vi "Generation Stream Control (Real 16 SPC).vi"(0 "data in":fxp<+/-,18,1>[](array[numeric])=[0.0, 0.0, 0.0, 0.0, 0.0, 0.0, 0.0, 0.0, 0.0, 0.0, 0.0, 0.0, 0.0, 0.0, 0.0, 0.0], 1 "input valid":bool, 2 "request state":T1, 3 "num samples":u64, 4 "initial padding":u64, 5 "final padding":u64, 7 "ready for output (T)":bool=TRUE, 8 "reset":bool, 9 "start trigger":bool) -> (11 "ready for start":bool, 12 "metadata":u64, 13 "ready for input":bool, 14 "data out":fxp<+/-,18,1>[](array[numeric]), 15 "output valid":bool, 16 "actual state":T1, 17 "samples transferred":u64)   [LabVIEW 2018, in "Streaming FPGA.lvlib"]
doc: "<B>General</B>\n\nThis VI controls the signal generation data flow with a state machine controller. This enables the control and monitoring of finite and continuous streams of data between nodes using 4-wire handshaking.\n\n<B>Signals</B>\n\nThe stream is controlled by the <B>request state</B>, <B>num samples</B>, <B>initial padding</B>, <B>final padding</B> and <B>start trigger</B> inputs. The stream is monitored by the <B>actual state</B>, <B>ready for start</B> and <B>samples transferred</B> outputs. In addition, <b>metadata</b> is available for publishing details about the form/function of the stream.\n\nThe upstream node can provide data on the <B>data in</B> input by setting the <B>input valid</B> input to true. The data provided on the <B>data in</B> input is accepted if the <B>input valid</B> input is true and the <B>ready for input</B> output was true in the previous cycle. If the <B>ready for input</B> output was false in the previous cycle, then the <B>data in</B> and <B>input valid</B> inputs are ignored in the current cycle.\n\nThe <B>output valid</B> output is set to true when data is available on the <B>data out</B> output. The downstream node should set the <B>ready for output</B> input to true when it is ready for data. If the <B>ready for output</B> input is true and the <B>output valid</B> output is also true, then the downstream node should accept the data provided on the <B>data out</B> output. If the <B>ready for output</B> input is false or if the <B>output valid</B> output is false, then the downstream should ignore the <B>data out</B> output.\n\n<B>Detailed Operation</B>\n\nThere are two signal generation modes: finite or continuous mode. Each time a signal generation is started <B>initial padding</B> number of padding samples are provided to the downstream node first, followed by <B>num samples</B> samples (in case of finite mode) or an unspecified number of samples (in case of continuous mode) provided by the upstream node. At the end of the signal generation <B>final padding</B> number of padding samples are provided to the downstream node. A finite signal generation can be started by transitioning the state machine from the Idle state to the Finite Transfer state. A continuous signal generation can be started by transitioning the state machine from the Idle state to the Continuous state. Transitioning from the Idle state to the Finite Transfer or Continuous state does not start the signal generation immediately, when transitioning into these states the state machine always waits for a start trigger before starting the generation. The state machine sets the <B>ready for start</B> output to true when it is waiting for a start trigger in the next cycle (otherwise this output is false), the start trigger can be provided on the <B>start trigger</B> input by setting this input to true. The <B>start trigger</B> to <B>output valid</B> delay is 1 cycle. Note that this VI assumes that the signal generation should be continuous: during the signal generation if the <B>ready for output</B> input is true, but no data can be provided to the downstream node, the state machine aborts the signal generation and enters the Error state.\n\n<B>samples transferred</B> is updated with the number of upstream node provided samples accepted by the downstream node in the current cycle, that is, this counter does not include the number of initial/final padding samples provided to the downstream node.\n\nIn finite mode the state machine enters the Done state once the signal generation is finished. In the Done state the samples transferred continues to be reported until the user requests that the state machine return to Idle. A signal generation can be aborted by entering the Cancel state. When entering the Cancel state, the final padding samples are still provided to the downstream node (in case the generation was started), then the state machine transitions to the Not Ready state, then it can transition into the Idle state.\n\nThis node uses an internal cache for storing samples provided by the upstream node. The upstream node is read in advance, samples stored in the internal cache are not flushed when a generation finishes, the samples remaining in the cache are returned during the next signal generation. The cache can be cleared by setting the <B>reset</B> input to true. This will also abort any ongoing signal generations but does not change the state of the internal state machine. In order to completely reset this VI set the <B>request state</B> input to Idle, set the <B>reset</B> input to true, wait until the <B>actual state</B> output indicates Idle, then set the <B>reset</B> input to false. Note that the upstream node is not read while this VI is in the Idle state.\n\n<b>States</b>\n\nThere are seven potential states for a stream defined by the Stream State.ctl typedef. All commanded states should be monitored from the controlling loop if it is important to ensure that the state is actually entered. The <B>request state</B> commands the stream into a state, and <B>actual state</B> reflects the current actual state.\n\nIdle - when the stream is ready to enter into an active state, it is in the Idle state. While it can be commanded directly to Idle from any state, it is advisable to do so with caution as samples abandoned in transfers may still need to be manually cleared out. It is generally safe to go directly from Done to Idle, and it is generally safe to request a transition from Not Ready to Idle. Other states may require further clean-up such as stopping/starting FIFOs or resetting other code under the command of the stream. Consider using Cancel instead (such as through the \"Stop Stream.vi\" in the host environment). While in Idle, <B>samples transferred</B> is reset to 0. \n\nFinite Transfer - Execute a transfer for the requested number of samples. Upon an orderly completion, this VI will automatically enter the Done state. If a stream underflows because the <B>ready for output</B> input is true, but no data can be provided to the downstream node, then the state machine enters the Error state.\n\nContinuous - Execute a transfer indefinitely. This state operates identically to the Finite Transfer state, but without regard to the <B>num samples</B> input.\n\nDone - In an orderly termination of a finite stream, the stream should end up here. At this point, <B>samples transferred</B> accurately reflects the terminal state of the transfer. The Done state should be exited by requesting Idle. Further active transfer modes (Finite or Continuous) will be ignored. This allows the host to distinguish between streams that are prematurely terminated (thus potentially requiring a flush of abandoned data) and ones that completed naturally.\n\nError - If the stream detects an unplanned interruption of the data, it enters the Error state. The only way to exit the Error state is to command the Generation Stream Control to Idle or Not Ready. When commanded to Idle or Not Ready, the Generation Stream Control advances first to Not Ready after the final padding samples are provided to the downstream node.\n\nNot Ready - In this state, the Generation Stream Control remains in the Not Ready state until the final padding samples are provided to the downstream node and the Generation Stream Control is commanded to Idle. This prevents starting a transfer in an obviously invalid state, and allows host control to wait until the not ready state is removed (such as by clearing out a FIFO under the streaming API's control).\n\nCancel - This state is indistinguishable from Error, but allows the controlling VI to know what condition caused the transfer to terminate."
uses:
  Streaming FPGA.lvlib
  <instrlib>/_niInstr/Streaming/v1/Common/Stream State.ctl
  <instrlib>/_niInstr/Streaming/v1/Common/niInstr Streaming v1 Common.lvlib
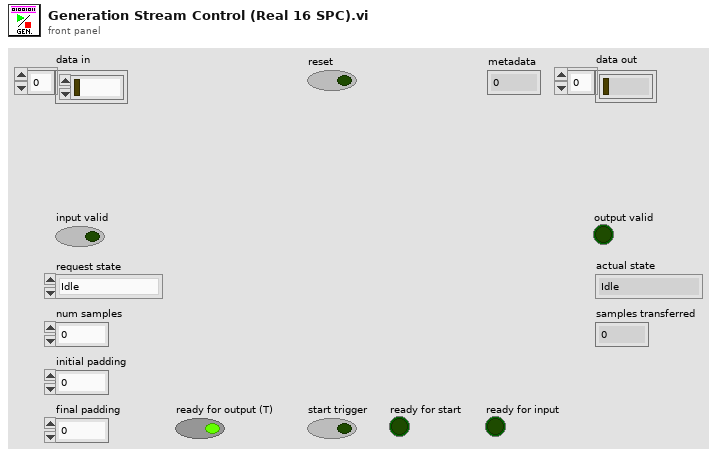
[diagram p1: front panel]
types:
  T1 = typedef "niInstr Streaming v1 Common.lvlib/Stream State.ctl" = enum8{"Idle", "Finite Transfer", "Continuous", "Done", "Error", "Not Ready", "Cancel"}
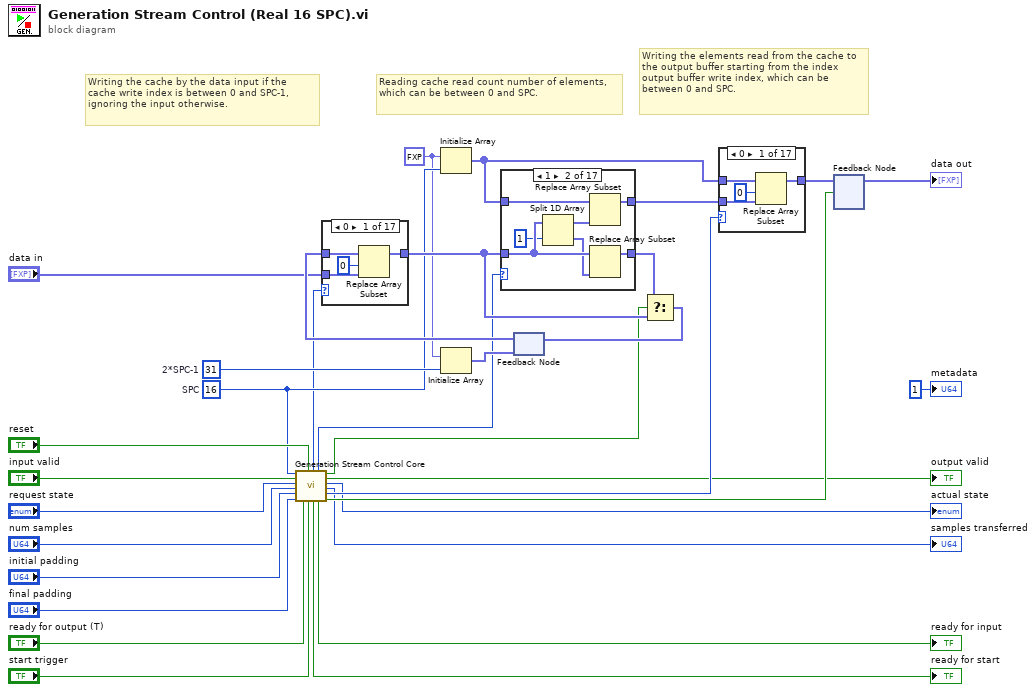
[diagram p0: block diagram]
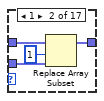
[diagram p2: hidden frame]
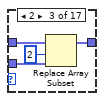
[diagram p3: hidden frame]
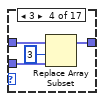
[diagram p4: hidden frame]
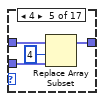
[diagram p5: hidden frame]
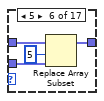
[diagram p6: hidden frame]
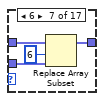
[diagram p7: hidden frame]
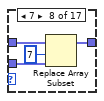
[diagram p8: hidden frame]
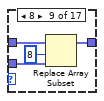
[diagram p9: hidden frame]
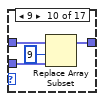
[diagram p10: hidden frame]
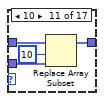
[diagram p11: hidden frame]
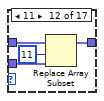
[diagram p12: hidden frame]
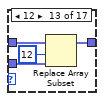
[diagram p13: hidden frame]
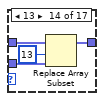
[diagram p14: hidden frame]
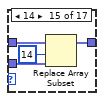
[diagram p15: hidden frame]
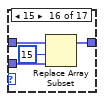
[diagram p16: hidden frame]
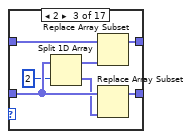
[diagram p19: hidden frame]
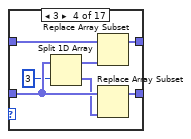
[diagram p20: hidden frame]
diagram:
  w1 = fxp<+/-,18,1> 0.0
  w20 = u8 16  # SPC
  w31 = u8 31  # 2*SPC-1
  # "Writing the elements read from the cache to the output buffer starting from the index output buffer write index, which can be between 0 and SPC."
  # "Reading cache read count number of elements, which can be between 0 and SPC."
  # "Writing the cache by the data input if the cache write index is between 0 and SPC-1, ignoring the input otherwise."
  n1 = call "Generation Stream Control Core.vi"("SPC"=w20, "input valid"="input valid", "request state"="request state", "num samples"="num samples", "initial padding"="initial padding", "final padding"="final padding", "ready for output (T)"="ready for output (T)", "reset"="reset", "start trigger"="start trigger") -> ("cache write index"=w19:u8, "ready for start"=→"ready for start":bool, "cache read count"=w18:u8, "ready for input"=→"ready for input":bool, "cache discard read elements"=w17:bool, "output valid"=→"output valid":bool, "actual state"=→"actual state":T1, "samples transferred"=→"samples transferred":u64, "output buffer write index"=w16:u8, "output buffer latch enable"=w15:bool)  [unwired: 1 in]
  n2 = Initialize Array(w1, w20) -> (w8:fxp<+/-,18,1>[])
  n3 = Initialize Array(w1, w31) -> (w30:fxp<+/-,18,1>[])
  n4 = feedback #1(w30) -> (w32:fxp<+/-,18,1>[])
  n5 = case shown="0" w19 {
    tunnel: w32 -> [w36 w40 w44 w48 w52 w56 w60 w64 w68 w72 w76 w80 w84 w88 w92 w96 w97]
    tunnel: "data in" -> [w35 w39 w43 w47 w51 w55 w59 w63 w67 w71 w75 w79 w83 w87 w91 w95 _]
    tunnel: [w33 w37 w41 w45 w49 w53 w57 w61 w65 w69 w73 w77 w81 w85 w89 w93 w97] -> w23
    frame 0 {
      n6 = Replace Array Subset(array=w36, new element=w35, index=0) -> (w33:fxp<+/-,18,1>[])
    }
    frame 1 {
      n7 = Replace Array Subset(array=w40, new element=w39, index=1) -> (w37:fxp<+/-,18,1>[])
    }
    frame 2 {
      n8 = Replace Array Subset(array=w44, new element=w43, index=2) -> (w41:fxp<+/-,18,1>[])
    }
    frame 3 {
      n9 = Replace Array Subset(array=w48, new element=w47, index=3) -> (w45:fxp<+/-,18,1>[])
    }
    frame 4 {
      n10 = Replace Array Subset(array=w52, new element=w51, index=4) -> (w49:fxp<+/-,18,1>[])
    }
    frame 5 {
      n11 = Replace Array Subset(array=w56, new element=w55, index=5) -> (w53:fxp<+/-,18,1>[])
    }
    frame 6 {
      n12 = Replace Array Subset(array=w60, new element=w59, index=6) -> (w57:fxp<+/-,18,1>[])
    }
    frame 7 {
      n13 = Replace Array Subset(array=w64, new element=w63, index=7) -> (w61:fxp<+/-,18,1>[])
    }
    frame 8 {
      n14 = Replace Array Subset(array=w68, new element=w67, index=8) -> (w65:fxp<+/-,18,1>[])
    }
    frame 9 {
      n15 = Replace Array Subset(array=w72, new element=w71, index=9) -> (w69:fxp<+/-,18,1>[])
    }
    frame 10 {
      n16 = Replace Array Subset(array=w76, new element=w75, index=10) -> (w73:fxp<+/-,18,1>[])
    }
    frame 11 {
      n17 = Replace Array Subset(array=w80, new element=w79, index=11) -> (w77:fxp<+/-,18,1>[])
    }
    frame 12 {
      n18 = Replace Array Subset(array=w84, new element=w83, index=12) -> (w81:fxp<+/-,18,1>[])
    }
    frame 13 {
      n19 = Replace Array Subset(array=w88, new element=w87, index=13) -> (w85:fxp<+/-,18,1>[])
    }
    frame 14 {
      n20 = Replace Array Subset(array=w92, new element=w91, index=14) -> (w89:fxp<+/-,18,1>[])
    }
    frame 15 {
      n21 = Replace Array Subset(array=w96, new element=w95, index=15) -> (w93:fxp<+/-,18,1>[])
    }
    frame Default {
    }
  }
  n22 = case shown="1" w18 {
    tunnel: w23 -> [w98 w106 w113 w120 w127 w134 w141 w148 w155 w162 w169 w176 w183 w190 w197 w204 w211]
    tunnel: [w98 w101 w108 w115 w122 w129 w136 w143 w150 w157 w164 w171 w178 w185 w192 w199 w206] -> w25
    tunnel: w8 -> [w99 w104 w111 w118 w125 w132 w139 w146 w153 w160 w167 w174 w181 w188 w195 w202 w209]
    tunnel: [w99 w102 w109 w116 w123 w130 w137 w144 w151 w158 w165 w172 w179 w186 w193 w200 w207] -> w28
    frame 0, Default {
    }
    frame 1 {
      n23 = Split 1D Array(array=w106, index=1) -> (first subarray=w103:fxp<+/-,18,1>[], second subarray=w105:fxp<+/-,18,1>[])
      n24 = Replace Array Subset(array=w104, new element=w103) -> (w102:fxp<+/-,18,1>[])  [unwired: 1 in]
      n25 = Replace Array Subset(array=w106, new element=w105) -> (w101:fxp<+/-,18,1>[])  [unwired: 1 in]
    }
    frame 2 {
      n26 = Split 1D Array(array=w113, index=2) -> (first subarray=w110:fxp<+/-,18,1>[], second subarray=w112:fxp<+/-,18,1>[])
      n27 = Replace Array Subset(array=w111, new element=w110) -> (w109:fxp<+/-,18,1>[])  [unwired: 1 in]
      n28 = Replace Array Subset(array=w113, new element=w112) -> (w108:fxp<+/-,18,1>[])  [unwired: 1 in]
    }
    frame 3 {
      n29 = Split 1D Array(array=w120, index=3) -> (first subarray=w117:fxp<+/-,18,1>[], second subarray=w119:fxp<+/-,18,1>[])
      n30 = Replace Array Subset(array=w118, new element=w117) -> (w116:fxp<+/-,18,1>[])  [unwired: 1 in]
      n31 = Replace Array Subset(array=w120, new element=w119) -> (w115:fxp<+/-,18,1>[])  [unwired: 1 in]
    }
    frame 4 {
      n32 = Split 1D Array(array=w127, index=4) -> (first subarray=w124:fxp<+/-,18,1>[], second subarray=w126:fxp<+/-,18,1>[])
      n33 = Replace Array Subset(array=w125, new element=w124) -> (w123:fxp<+/-,18,1>[])  [unwired: 1 in]
      n34 = Replace Array Subset(array=w127, new element=w126) -> (w122:fxp<+/-,18,1>[])  [unwired: 1 in]
    }
    frame 5 {
      n35 = Split 1D Array(array=w134, index=5) -> (first subarray=w131:fxp<+/-,18,1>[], second subarray=w133:fxp<+/-,18,1>[])
      n36 = Replace Array Subset(array=w132, new element=w131) -> (w130:fxp<+/-,18,1>[])  [unwired: 1 in]
      n37 = Replace Array Subset(array=w134, new element=w133) -> (w129:fxp<+/-,18,1>[])  [unwired: 1 in]
    }
    frame 6 {
      n38 = Split 1D Array(array=w141, index=6) -> (first subarray=w138:fxp<+/-,18,1>[], second subarray=w140:fxp<+/-,18,1>[])
      n39 = Replace Array Subset(array=w139, new element=w138) -> (w137:fxp<+/-,18,1>[])  [unwired: 1 in]
      n40 = Replace Array Subset(array=w141, new element=w140) -> (w136:fxp<+/-,18,1>[])  [unwired: 1 in]
    }
    frame 7 {
      n41 = Split 1D Array(array=w148, index=7) -> (first subarray=w145:fxp<+/-,18,1>[], second subarray=w147:fxp<+/-,18,1>[])
      n42 = Replace Array Subset(array=w146, new element=w145) -> (w144:fxp<+/-,18,1>[])  [unwired: 1 in]
      n43 = Replace Array Subset(array=w148, new element=w147) -> (w143:fxp<+/-,18,1>[])  [unwired: 1 in]
    }
    frame 8 {
      n44 = Split 1D Array(array=w155, index=8) -> (first subarray=w152:fxp<+/-,18,1>[], second subarray=w154:fxp<+/-,18,1>[])
      n45 = Replace Array Subset(array=w153, new element=w152) -> (w151:fxp<+/-,18,1>[])  [unwired: 1 in]
      n46 = Replace Array Subset(array=w155, new element=w154) -> (w150:fxp<+/-,18,1>[])  [unwired: 1 in]
    }
    frame 9 {
      n47 = Split 1D Array(array=w162, index=9) -> (first subarray=w159:fxp<+/-,18,1>[], second subarray=w161:fxp<+/-,18,1>[])
      n48 = Replace Array Subset(array=w160, new element=w159) -> (w158:fxp<+/-,18,1>[])  [unwired: 1 in]
      n49 = Replace Array Subset(array=w162, new element=w161) -> (w157:fxp<+/-,18,1>[])  [unwired: 1 in]
    }
    frame 10 {
      n50 = Split 1D Array(array=w169, index=10) -> (first subarray=w166:fxp<+/-,18,1>[], second subarray=w168:fxp<+/-,18,1>[])
      n51 = Replace Array Subset(array=w167, new element=w166) -> (w165:fxp<+/-,18,1>[])  [unwired: 1 in]
      n52 = Replace Array Subset(array=w169, new element=w168) -> (w164:fxp<+/-,18,1>[])  [unwired: 1 in]
    }
    frame 11 {
      n53 = Split 1D Array(array=w176, index=11) -> (first subarray=w173:fxp<+/-,18,1>[], second subarray=w175:fxp<+/-,18,1>[])
      n54 = Replace Array Subset(array=w174, new element=w173) -> (w172:fxp<+/-,18,1>[])  [unwired: 1 in]
      n55 = Replace Array Subset(array=w176, new element=w175) -> (w171:fxp<+/-,18,1>[])  [unwired: 1 in]
    }
    frame 12 {
      n56 = Split 1D Array(array=w183, index=12) -> (first subarray=w180:fxp<+/-,18,1>[], second subarray=w182:fxp<+/-,18,1>[])
      n57 = Replace Array Subset(array=w181, new element=w180) -> (w179:fxp<+/-,18,1>[])  [unwired: 1 in]
      n58 = Replace Array Subset(array=w183, new element=w182) -> (w178:fxp<+/-,18,1>[])  [unwired: 1 in]
    }
    frame 13 {
      n59 = Split 1D Array(array=w190, index=13) -> (first subarray=w187:fxp<+/-,18,1>[], second subarray=w189:fxp<+/-,18,1>[])
      n60 = Replace Array Subset(array=w188, new element=w187) -> (w186:fxp<+/-,18,1>[])  [unwired: 1 in]
      n61 = Replace Array Subset(array=w190, new element=w189) -> (w185:fxp<+/-,18,1>[])  [unwired: 1 in]
    }
    frame 14 {
      n62 = Split 1D Array(array=w197, index=14) -> (first subarray=w194:fxp<+/-,18,1>[], second subarray=w196:fxp<+/-,18,1>[])
      n63 = Replace Array Subset(array=w195, new element=w194) -> (w193:fxp<+/-,18,1>[])  [unwired: 1 in]
      n64 = Replace Array Subset(array=w197, new element=w196) -> (w192:fxp<+/-,18,1>[])  [unwired: 1 in]
    }
    frame 15 {
      n65 = Split 1D Array(array=w204, index=15) -> (first subarray=w201:fxp<+/-,18,1>[], second subarray=w203:fxp<+/-,18,1>[])
      n66 = Replace Array Subset(array=w202, new element=w201) -> (w200:fxp<+/-,18,1>[])  [unwired: 1 in]
      n67 = Replace Array Subset(array=w204, new element=w203) -> (w199:fxp<+/-,18,1>[])  [unwired: 1 in]
    }
    frame 16 {
      n68 = Split 1D Array(array=w211, index=16) -> (first subarray=w208:fxp<+/-,18,1>[], second subarray=w210:fxp<+/-,18,1>[])
      n69 = Replace Array Subset(array=w209, new element=w208) -> (w207:fxp<+/-,18,1>[])  [unwired: 1 in]
      n70 = Replace Array Subset(array=w211, new element=w210) -> (w206:fxp<+/-,18,1>[])  [unwired: 1 in]
    }
  }
  n71 = Select(t=w25, s=w17, f=w23) -> (s? t:f=w24:fxp<+/-,18,1>[])
  n72 = feedback-in #1(w24) -> ()
  n73 = case shown="0" w16 {
    tunnel: w8 -> [w215 w219 w223 w227 w231 w235 w239 w243 w247 w251 w255 w259 w263 w267 w271 w275 w276]
    tunnel: w28 -> [w214 w218 w222 w226 w230 w234 w238 w242 w246 w250 w254 w258 w262 w266 w270 w274 _]
    tunnel: [w212 w216 w220 w224 w228 w232 w236 w240 w244 w248 w252 w256 w260 w264 w268 w272 w276] -> w27
    frame 0 {
      n74 = Replace Array Subset(array=w215, new element=w214, index=0) -> (w212:fxp<+/-,18,1>[])
    }
    frame 1 {
      n75 = Replace Array Subset(array=w219, new element=w218, index=1) -> (w216:fxp<+/-,18,1>[])
    }
    frame 2 {
      n76 = Replace Array Subset(array=w223, new element=w222, index=2) -> (w220:fxp<+/-,18,1>[])
    }
    frame 3 {
      n77 = Replace Array Subset(array=w227, new element=w226, index=3) -> (w224:fxp<+/-,18,1>[])
    }
    frame 4 {
      n78 = Replace Array Subset(array=w231, new element=w230, index=4) -> (w228:fxp<+/-,18,1>[])
    }
    frame 5 {
      n79 = Replace Array Subset(array=w235, new element=w234, index=5) -> (w232:fxp<+/-,18,1>[])
    }
    frame 6 {
      n80 = Replace Array Subset(array=w239, new element=w238, index=6) -> (w236:fxp<+/-,18,1>[])
    }
    frame 7 {
      n81 = Replace Array Subset(array=w243, new element=w242, index=7) -> (w240:fxp<+/-,18,1>[])
    }
    frame 8 {
      n82 = Replace Array Subset(array=w247, new element=w246, index=8) -> (w244:fxp<+/-,18,1>[])
    }
    frame 9 {
      n83 = Replace Array Subset(array=w251, new element=w250, index=9) -> (w248:fxp<+/-,18,1>[])
    }
    frame 10 {
      n84 = Replace Array Subset(array=w255, new element=w254, index=10) -> (w252:fxp<+/-,18,1>[])
    }
    frame 11 {
      n85 = Replace Array Subset(array=w259, new element=w258, index=11) -> (w256:fxp<+/-,18,1>[])
    }
    frame 12 {
      n86 = Replace Array Subset(array=w263, new element=w262, index=12) -> (w260:fxp<+/-,18,1>[])
    }
    frame 13 {
      n87 = Replace Array Subset(array=w267, new element=w266, index=13) -> (w264:fxp<+/-,18,1>[])
    }
    frame 14 {
      n88 = Replace Array Subset(array=w271, new element=w270, index=14) -> (w268:fxp<+/-,18,1>[])
    }
    frame 15 {
      n89 = Replace Array Subset(array=w275, new element=w274, index=15) -> (w272:fxp<+/-,18,1>[])
    }
    frame 16, Default {
    }
  }
  n90 = feedback-in #2(w27, w15) -> ()
  n91 = feedback #2() -> (→"data out":fxp<+/-,18,1>[])  [unwired: 1 in]
  "metadata" <- u64 1 ("metadata")
